vi "Bamocar Serial.vi"(8 "Error In":errorcluster, 9 "Value to Write":string="0FA0", 11 "Command":enum16{"Write/Read", "Write", "Read"}(ring)=enum."Read") -> (0 "Error Out":errorcluster={"status"=TRUE, "code"=-1073807339, "source"="VISA Read in Bamocar Main.vi"}, 3 "Decimal":u32)   [LabVIEW 2017]
uses:
  <vilib>/Instr/_visa.llb/VISA Configure Serial Port (Instr).vi
panel:
  in  "Register":u16(ring) items=["Drive Enable"=81]
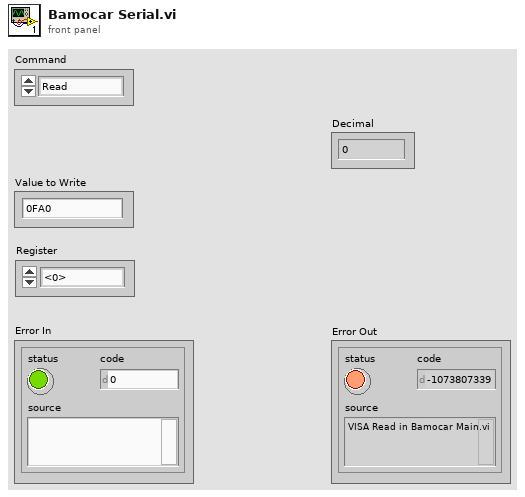
[diagram p1: front panel]
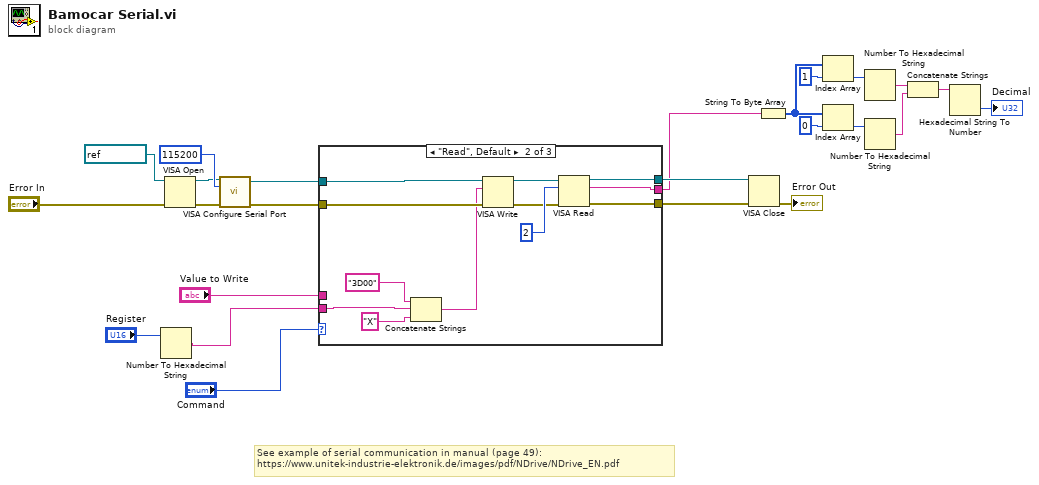
[diagram p0: block diagram]
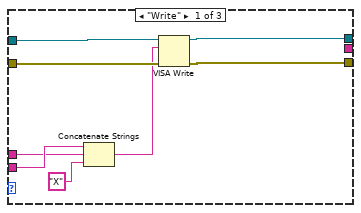
[diagram p2: hidden frame]
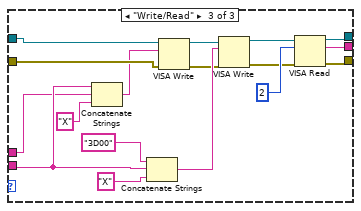
[diagram p3: hidden frame]
diagram:
  # "See example of serial communication in manual (page 49):\nhttps://www.unitek-industrie-elektronik.de/images/pdf/NDrive/NDrive_EN.pdf"
  n1 = Number To Hexadecimal String(2:"Register") -> (0:w1:string)  [unwired: 1 in]
  n2 = VISA Open(error in (no error)="Error In", VISA resource name=refnum<visa-resource-name> "COM4") -> (VISA resource name=w22:refnum<visa-resource-name>, error out=w23:errorcluster)  [unwired: 3 in]
  n3 = call-poly "VISA Configure Serial Port"("VISA resource name"=w22, "baud rate (9600)"=u32 115200, "error in (no error)"=w23) -> ("VISA resource name out"=w6:refnum<visa-resource-name>, "error out"=w7:errorcluster)  [unwired: 11 in]
  n4 = case shown="\"Read\", Default" "Command" {
    tunnel: w1 -> [w32 w43 w46]
    tunnel: "Value to Write" -> [w31 _ w45]
    tunnel: w7 -> [w28 w41 w50]
    tunnel: w6 -> [w29 w39 w49]
    tunnel: [w26 w35 w55] -> w5
    tunnel: [w25 w34 w54] -> w4
    tunnel: [_ w33 w53] -> w3
    frame "Write" {
      n5 = Concatenate Strings(w32, w31, "X" ("string")) -> (w27:string)
      n6 = VISA Write(VISA resource name=w29, write buffer=w27, error in (no error)=w28) -> (VISA resource name out=w25:refnum<visa-resource-name>, error out=w26:errorcluster)  [unwired: 1 out]
    }
    frame "Read", Default {
      n7 = Concatenate Strings("3D00" ("string"), w43, "X" ("string")) -> (w40:string)
      n8 = VISA Write(VISA resource name=w39, write buffer=w40, error in (no error)=w41) -> (VISA resource name out=w36:refnum<visa-resource-name>, error out=w37:errorcluster)  [unwired: 1 out]
      n9 = VISA Read(VISA resource name=w36, byte count=u32 2, error in (no error)=w37) -> (VISA resource name out=w34:refnum<visa-resource-name>, read buffer=w33:string, error out=w35:errorcluster)  [unwired: 1 out]
    }
    frame "Write/Read" {
      n10 = Concatenate Strings(w46, w45, "X" ("string")) -> (w47:string)
      n11 = Concatenate Strings("3D00" ("string"), w46, "X" ("string")) -> (w59:string)
      n12 = VISA Write(VISA resource name=w49, write buffer=w47, error in (no error)=w50) -> (VISA resource name out=w51:refnum<visa-resource-name>, error out=w52:errorcluster)  [unwired: 1 out]
      n13 = VISA Write(VISA resource name=w51, write buffer=w59, error in (no error)=w52) -> (VISA resource name out=w56:refnum<visa-resource-name>, error out=w57:errorcluster)  [unwired: 1 out]
      n14 = VISA Read(VISA resource name=w56, byte count=u32 2, error in (no error)=w57) -> (VISA resource name out=w54:refnum<visa-resource-name>, read buffer=w53:string, error out=w55:errorcluster)  [unwired: 1 out]
    }
  }
  n15 = VISA Close(VISA resource name=w4, error in (no error)=w5) -> (error out=→"Error Out":errorcluster)
  n16 = String To Byte Array(string=w3) -> (unsigned byte array=w14:u8[])
  n17 = Index Array(array=w14, index=1) -> (element=w16:u8)
  n18 = Index Array(array=w14, index=0) -> (element=w13:u8)
  n19 = Number To Hexadecimal String(2:w16) -> (0:w12:string)  [unwired: 1 in]
  n20 = Number To Hexadecimal String(2:w13) -> (0:w9:string)  [unwired: 1 in]
  n21 = Concatenate Strings(w12, w9) -> (w11:string)
  n22 = Hexadecimal String To Number(string=w11) -> (number=→"Decimal":u32)  [unwired: 2 in, 1 out]
